vi "KBDConnectMoveTo.vi"() -> ()   [LabVIEW 2015]
uses:
  C:/Users/fmovagharnemati/OneDrive - THORLABS Inc/Desktop/github/KBD101/Thorlabs.MotionControl.Controls.dll
  github/KBD101/Thorlabs.MotionControl.Controls.dll
  C:/Users/fmovagharnemati/OneDrive - THORLABS Inc/Desktop/github/KBD101/Thorlabs.MotionControl.KCube.BrushlessMotorCLI.dll
  github/KBD101/Thorlabs.MotionControl.KCube.BrushlessMotorCLI.dll
panel:
  out "Device Busy":bool
  in  "Move To Position":bool
  in  "Disconnect":bool
  out "Device Needs Homing":bool
  in  "position":dbl
  in  "SerialNumber":string
  in  "KCubeBrushlessControl":refnum<k24>(container)
  # "Thorlabs Hardware: KBD - K-Cube Brushless DC Servo Driver\nhttps://www.thorlabs.com/thorproduct.cfm?partnumber=KBD101\n\nDescription: This VI will enable you to communicate with KBD101  to control  Brushless Stages & Actuators. The VI will first connect and initialize the device, home it, and await user command to move to a specified location.\n\nInstructions: \n1) Connect your KBD101  device to your PC & power the device, ensuring your stage/actutator is connected. For full device setup, the device product manual can be found on our website here. -https://www.thorlabs.com/thorproduct.cfm?partnumber=KBD101\n2) Enter the device serial number below.\n3) Ensure the device move path is clear for homing.\n4) Click 'Run' in the LabVIEW Toolbar which will attempt a connection, and a home command in that order.\n5) Await for device to be be available, and to have finished homing.\n6) Input desired movement position, and press 'Move To Position'.\n7) To end the Program click 'STOP'."
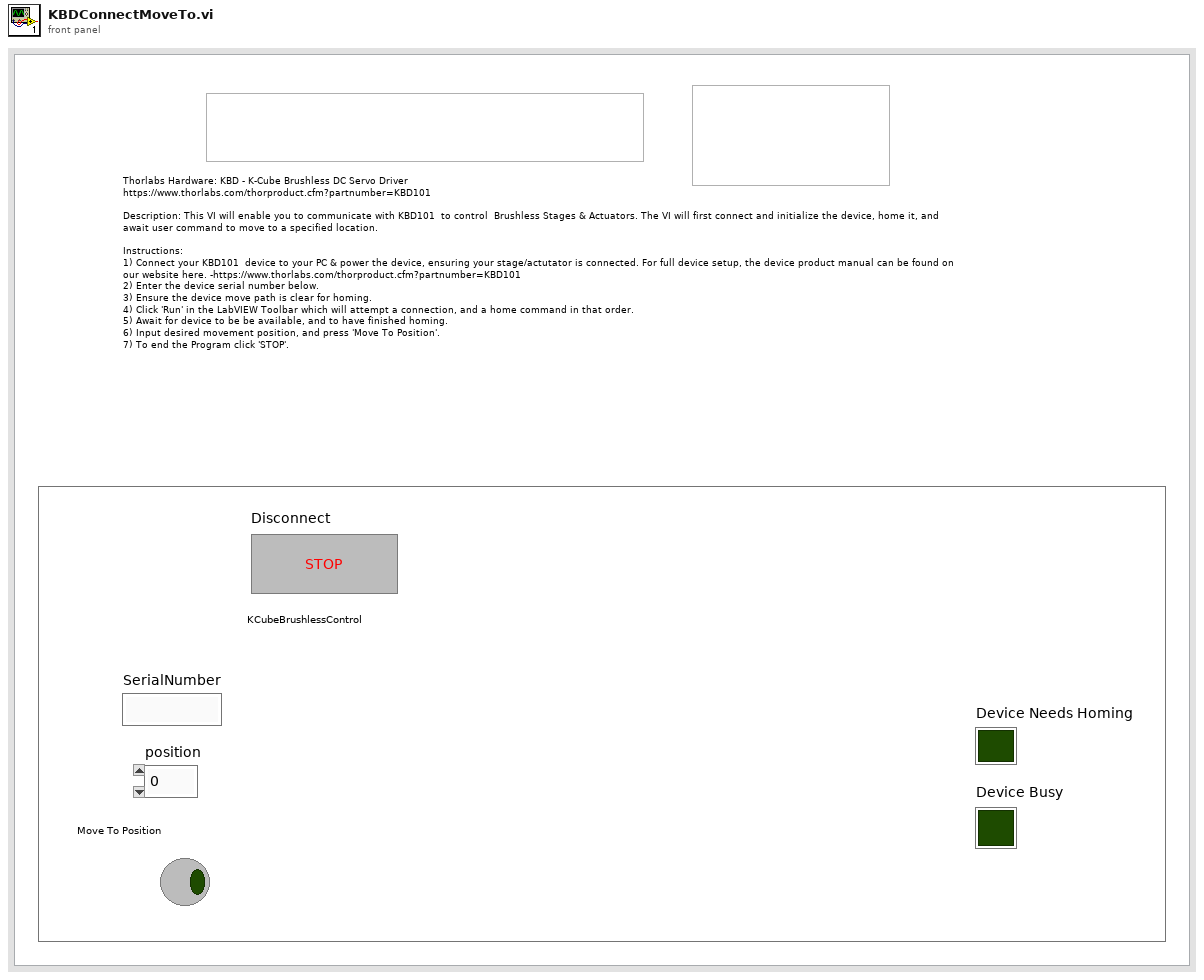
[diagram p1: front panel]
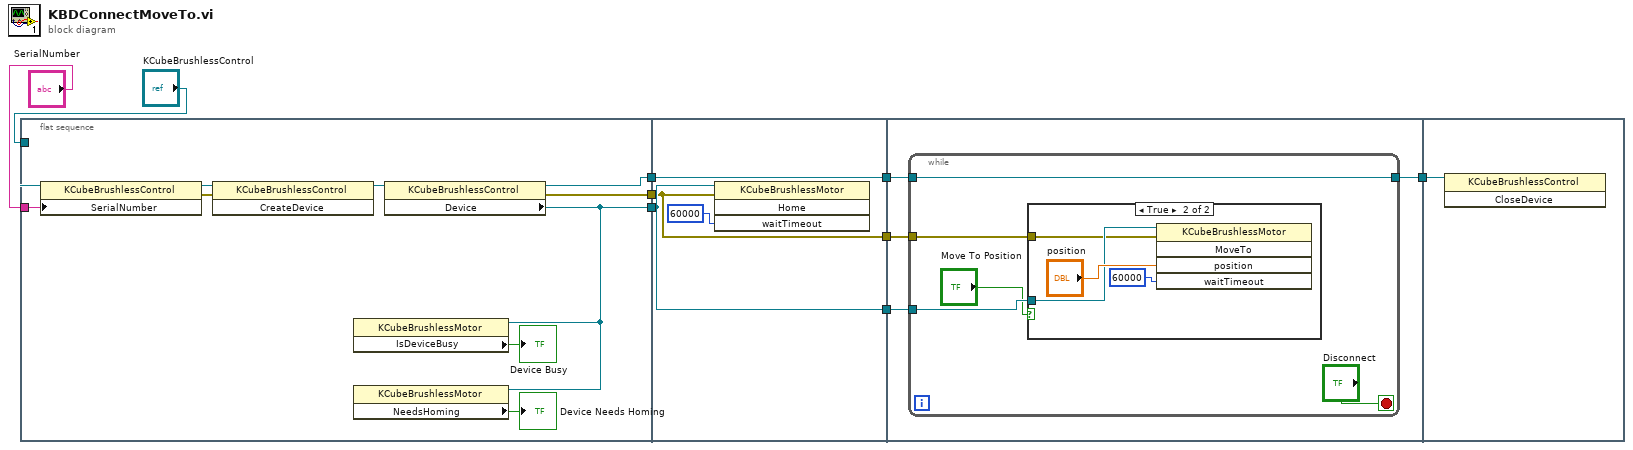
[diagram p0: block diagram]
diagram:
  n1 = flat-sequence {
    tunnel: "KCubeBrushlessControl" -> [w18]
    tunnel: "SerialNumber" -> [w16]
    tunnel: [w13] -> w7
    tunnel: [w12] -> w6
    tunnel: [w11] -> w5
    tunnel: w7 -> [w21]
    tunnel: w6 -> [w20]
    tunnel: w5 -> [w22]
    tunnel: [w22] -> w4
    tunnel: [w21] -> w3
    tunnel: [w20] -> w2
    tunnel: w4 -> [w27]
    tunnel: w3 -> [w26]
    tunnel: w2 -> [w25]
    tunnel: [w24] -> w1
    tunnel: w1 -> [w37]
    frame #0 {
      n2 = property class="KCubeBrushlessControl"(reference=w18, "SerialNumber"=w16) -> (reference out=w19:refnum<k24>, error out=w17:errorcluster)  [unwired: 1 in]
      n3 = invoke class="KCubeBrushlessControl" method="CreateDevice"(reference=w19, error in=w17) -> (reference out=w15:refnum<k24>)  [unwired: 1 in, 2 out]
      n4 = property class="KCubeBrushlessControl"(reference=w15) -> (reference out=w11:refnum<k24>, error out=w12:errorcluster, "Device"=w13:refnum<k24>)  [unwired: 1 in]
      n5 = property class="KCubeBrushlessMotor"(reference=w13) -> ("IsDeviceBusy"=→"Device Busy":bool)  [unwired: 1 in, 2 out]
      n6 = property class="KCubeBrushlessMotor"(reference=w13) -> ("NeedsHoming"=→"Device Needs Homing":bool)  [unwired: 1 in, 2 out]
    }
    frame #1 {
      n7 = invoke class="KCubeBrushlessMotor" method="Home"(reference=w21, error in=w20, "waitTimeout"=60000) -> ()  [unwired: 1 in, 4 out]
    }
    frame #2 {
      n8 = while {
        tunnel: [w32] -> w24
        tunnel: w27 -> [w32]
        tunnel: w26 -> [w31]
        tunnel: w25 -> [w30]
        stop <- "Disconnect" stop-if-true
        n9 = case shown="True" "Move To Position" {
          tunnel: w31 -> [_ w34]
          tunnel: w30 -> [_ w33]
          frame False {
          }
          frame True {
            n10 = invoke class="KCubeBrushlessMotor" method="MoveTo"(reference=w34, error in=w33, "position"="position", "waitTimeout"=60000) -> ()  [unwired: 1 in, 5 out]
          }
        }
      }
    }
    frame #3 {
      n11 = invoke class="KCubeBrushlessControl" method="CloseDevice"(reference=w37) -> ()  [unwired: 2 in, 3 out]
    }
  }
